vi "Config Write Channels.vi"(8 "error in (no error)":errorcluster, 10 "Discrete Inputs":T2[](array[typedef]), 11 "Refnum in":T1) -> (0 "error out":errorcluster, 3 "Refnum out":T1)   [LabVIEW 2015, in "Modbus Master System Explorer.lvlib"]
uses:
  Modbus Master System Explorer.lvlib
  <vilib>/Utility/config.llb/Config Data RefNum.ctl
  Shared/Controls/Data Model/Channel.ctl
  Modbus Type.ctl
  <vilib>/NI Veristand/Custom Device API/Custom Device Channel Type.ctl
  Shared/Controls/Data Model/Mapping.ctl
  Shared/Controls/Data Model/DataType.ctl
  <vilib>/NI Veristand/Custom Device API/Custom Device Item Ref.ctl
  <vilib>/Utility/config.llb/Write Key (String).vi
  <vilib>/Utility/config.llb/Write Key (U32).vi
  <vilib>/Utility/config.llb/NI_LVConfig.lvlib
  Shared/Modbus Master Shared.lvlib
  <vilib>/NI VeriStand/Custom Device API/Custom Device API.lvlib
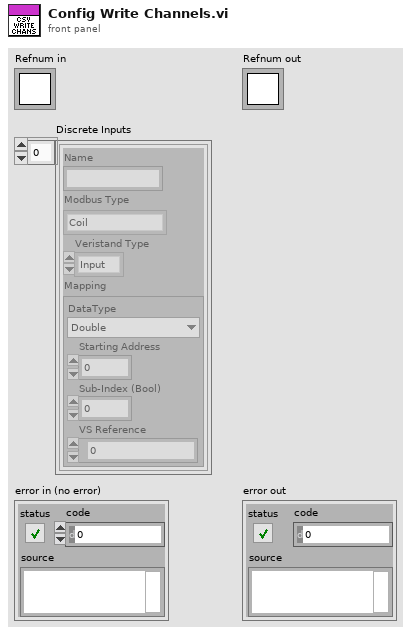
[diagram p1: front panel]
types:
  T1 = typedef "NI_LVConfig.lvlib/Config Data RefNum.ctl" = refnum<k1>
  T2 = typedef "Modbus Master Shared.lvlib/Channel.ctl" = cluster{"Name":string, "Modbus Type":T3, "Veristand Type":T4, "Mapping":T5}
  T3 = typedef "Modbus Master Shared.lvlib/Modbus Type.ctl" = enum16{"Coil", "Discrete Input", "Holding Register", "Input Register"}
  T4 = typedef "Custom Device API.lvlib/Custom Device Channel Type.ctl" = enum16{"Input", "Output"}
  T5 = typedef "Modbus Master Shared.lvlib/Mapping.ctl" = cluster{"DataType":T6, "Starting Address":u16, "Sub-Index (Bool)":u16, "VS Reference":T7}
  T6 = typedef "Modbus Master Shared.lvlib/DataType.ctl" = enum16{"Double", "Single", "I64", "I32", "I16", "I8", "U64", "U32", "U16", "U8", "Boolean"}
  T7 = typedef "Custom Device API.lvlib/Custom Device Item Ref.ctl" = u64
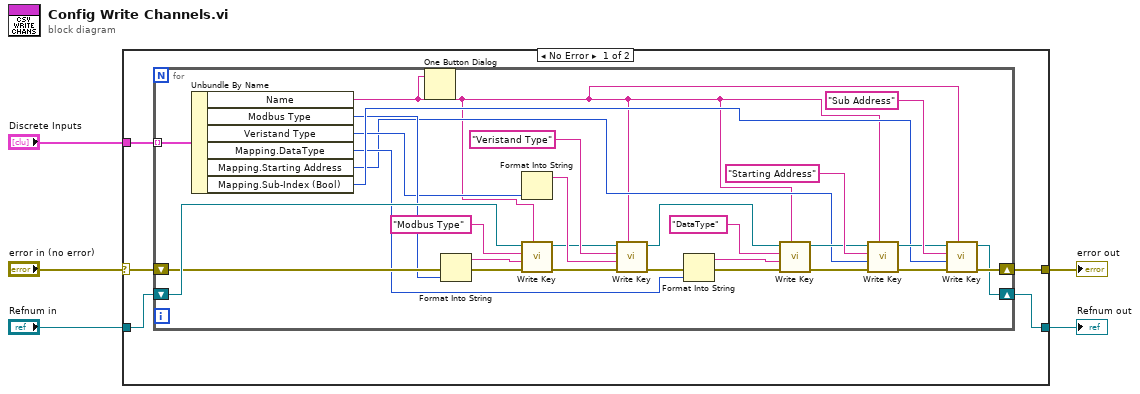
[diagram p0: block diagram]
diagram:
  n1 = case shown="No Error" "error in (no error)" {
    selector: "error in (no error)" -> [w10 w40]
    tunnel: "Refnum in" -> [w9 w41]
    tunnel: "Discrete Inputs" -> [w8 _]
    tunnel: [w7 w40] -> w2
    tunnel: [w6 w41] -> w1
    frame No Error {
      n2 = for {
        shift-right: [w14] -> w7
        shift-left: w10 -> [w27]
        tunnel: w8 -> [w39] mode=indexing
        shift-right: [w13] -> w6
        shift-left: w9 -> [w30]
        n3 = Unbundle By Name(w39) -> ("Name"=w11:string, "Modbus Type"=w26:T3, "Veristand Type"=w24:T4, "Mapping.DataType"=w20:T6, "Mapping.Starting Address"=w12:u16, "Mapping.Sub-Index (Bool)"=w33:u16)
        n4 = One Button Dialog(message=w11) -> ()  [unwired: 1 in, 1 out]
        n5 = Format Into String(error in=w27, w26) -> (resulting string=w29:string, error out=w28:errorcluster)  [unwired: 2 in]
        n6 = Format Into String(w24) -> (resulting string=w23:string)  [unwired: 3 in, 1 out]
        n7 = call-poly <vilib>:"Write Key.vi"("section"=w11, "error in (no error)"=w28, "value"=w29, "key"="Modbus Type", "refnum"=w30) -> ("error out"=w22:errorcluster, "refnum out"=w21:T1)  [unwired: 4 in, 1 out]
        n8 = call-poly <vilib>:"Write Key.vi"("section"=w11, "error in (no error)"=w22, "value"=w23, "key"="Veristand Type", "refnum"=w21) -> ("error out"=w17:errorcluster, "refnum out"=w19:T1)  [unwired: 4 in, 1 out]
        n9 = Format Into String(error in=w17, w20) -> (resulting string=w31:string, error out=w16:errorcluster)  [unwired: 2 in]
        n10 = call-poly <vilib>:"Write Key.vi"("section"=w11, "error in (no error)"=w16, "value"=w31, "key"="DataType", "refnum"=w19) -> ("error out"=w15:errorcluster, "refnum out"=w18:T1)  [unwired: 4 in, 1 out]
        n11 = call-poly <vilib>:"Write Key.vi"("section"=w11, "error in (no error)"=w15, "value"=w12, "key"="Starting Address", "refnum"=w18) -> ("error out"=w35:errorcluster, "refnum out"=w34:T1)  [unwired: 4 in, 1 out]
        n12 = call-poly <vilib>:"Write Key.vi"("section"=w11, "error in (no error)"=w35, "value"=w33, "key"="Sub Address", "refnum"=w34) -> ("error out"=w14:errorcluster, "refnum out"=w13:T1)  [unwired: 4 in, 1 out]
      }
    }
    frame Error {
    }
  }
  "error out" <- w2
  "Refnum out" <- w1
